vi "Write SA Parameters.vi"(8 "error in (no error)":errorcluster, 10 "SA Parameters":T1, 11 "Skyworks Spur Test in":refnum<class "Skyworks Spur Test.lvclass">) -> (0 "error out":errorcluster, 3 "Skyworks Spur Test out":refnum<class "Skyworks Spur Test.lvclass">)   [LabVIEW 2018, in "Skyworks Spur Test.lvlib" / "Skyworks Spur Test.lvclass"]
uses:
  Skyworks Spur Test.lvclass
  Controls/SA Parameters.ctl
  Skyworks Spur Test.lvclass/Skyworks Spur Test.ctl
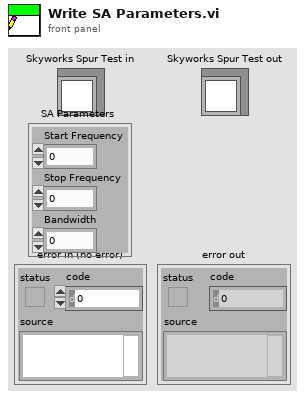
[diagram p1: front panel]
types:
  T1 = typedef "Skyworks Spur Test.lvlib/Skyworks Spur Test.lvclass/SA Parameters.ctl" = cluster{"Start Frequency":dbl, "Stop Frequency":dbl, "Bandwidth":dbl}
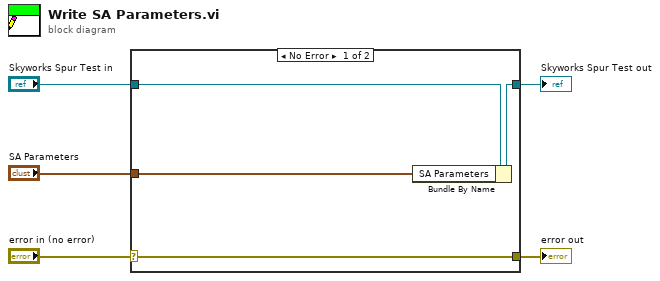
[diagram p0: block diagram]
diagram:
  n1 = case shown="No Error" "error in (no error)" {
    selector: "error in (no error)" -> [w9 w10]
    tunnel: [w9 w10] -> w4
    tunnel: [w7 w11] -> w2
    tunnel: "Skyworks Spur Test in" -> [w8 w11]
    tunnel: "SA Parameters" -> [w6 _]
    frame No Error {
      n2 = Bundle By Name(cluster=w8, "SA Parameters"=w6) -> (w7:refnum<class "Skyworks Spur Test.lvclass">)
    }
    frame Error {
    }
  }
  "error out" <- w4
  "Skyworks Spur Test out" <- w2
